vi "Temp.vi"() -> ()   [LabVIEW 2009]
uses:
  <vilib>/Platform/TimedLoop/XDataNode/XDataNode.xnode
  <vilib>/Platform/TimedLoop/XDataNode/loadlvalarms.vi
  <vilib>/Platform/TimedLoop/XDataNode/timing_clust.ctl
  <vilib>/Platform/TimedLoop/XDataNode/nitl_modes.ctl
  <vilib>/Platform/TimedLoop/XDataNode/wakeup.ctl
  <vilib>/Platform/TimedLoop/XDataNode/XDNodeRunTimeDep.lvlib
  <vilib>/Analysis/NI_AALBase.lvlib
  <vilib>/Analysis/NI_AALPro.lvlib
panel:
  out "time":dbl[](array[numeric])
  out "bearing":dbl[](array[numeric])
  out "XY Graph":cluster{dbl[], dbl[]}(graph)
  in  "Buffer Dimension":i32=10
  out "Iteration Duration 2":i64
  out "appended array":dbl[](array[numeric])
  in  "Simulate?":bool=TRUE
  out "Iteration Duration":i64=996
  in  "Prediction Time (s)":dbl=1.0
  out "Target Bearing":dbl
  in  "Sampling Time":dbl[](array[numeric])
  in  "Bearing History":dbl[](array[numeric])
  out "Bearing Sample":dbl=191.29579607174375 format="%0.2f"
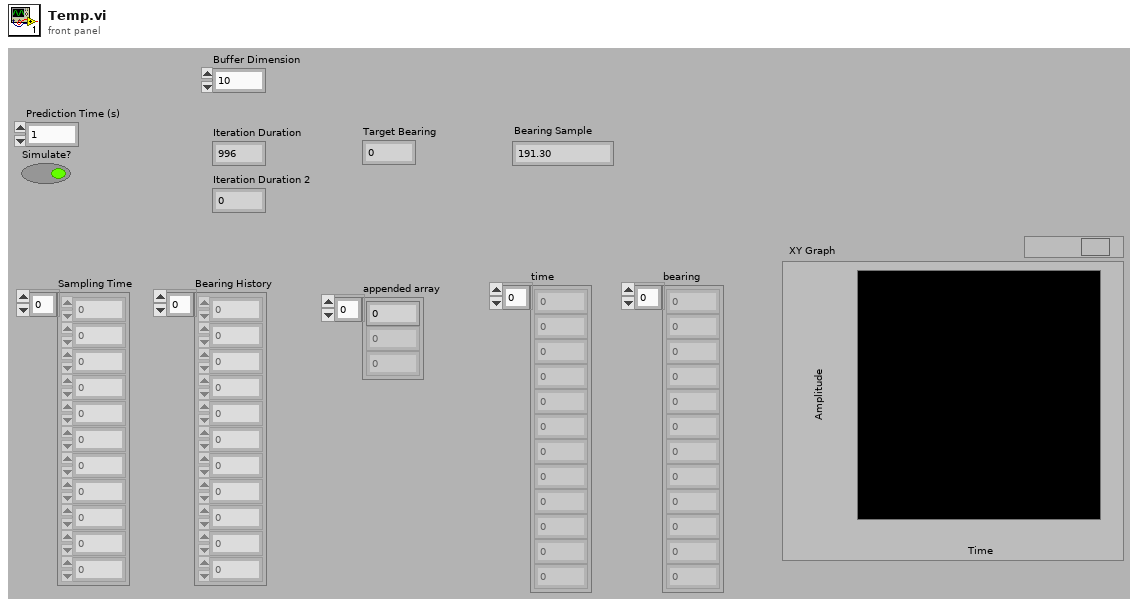
[diagram p1: front panel]
types:
  T1 = typedef "XDNodeRunTimeDep.lvlib/timing_clust.ctl" = cluster{"Expected End [f-1]":u64, "Actual End [f-1]":u64, "Finished Late? [f-1]":bool, "Expected End [i-1]":u64, "Actual End [i-1]":u64, "Finished Late? [i-1]":bool, "Expected Start [i]":u64, "Actual Start [i]":u64, "Expected Start [f]":u64, "Actual Start [f]":u64, "Source Name":string, "Structure Name":string, "Period":i64, "Deadline":i64, "Offset":i64, "Start":i64, "Priority":i32, "Timeout":i32, "Mode":T2, "Wakeup Reason":T3, "Error":errorcluster, "Source Type":string, "Secondary Source Type":string, "Global End Time":u64, "Global Start Time":u64, "Frame Duration":u64, "Iteration Duration":u64, "Assigned CPU":i32, "I/O Scan Engine Mode":u32}
  T2 = typedef "XDNodeRunTimeDep.lvlib/nitl_modes.ctl" = enum32{"No Change", "Process missed periods, maintain original phase", "Discard missed periods, maintain original phase", "Process missed periods, ignore original phase", "Discard missed periods, ignore original phase"}
  T3 = typedef "XDNodeRunTimeDep.lvlib/wakeup.ctl" = enum32{"Normal", "Aborted", "Asynchronous wakeup", "Timing source error", "Timed loop error", "Timeout"}
  T4 = cluster{"Sampling Time":dbl[], "Bearing History":dbl[]}
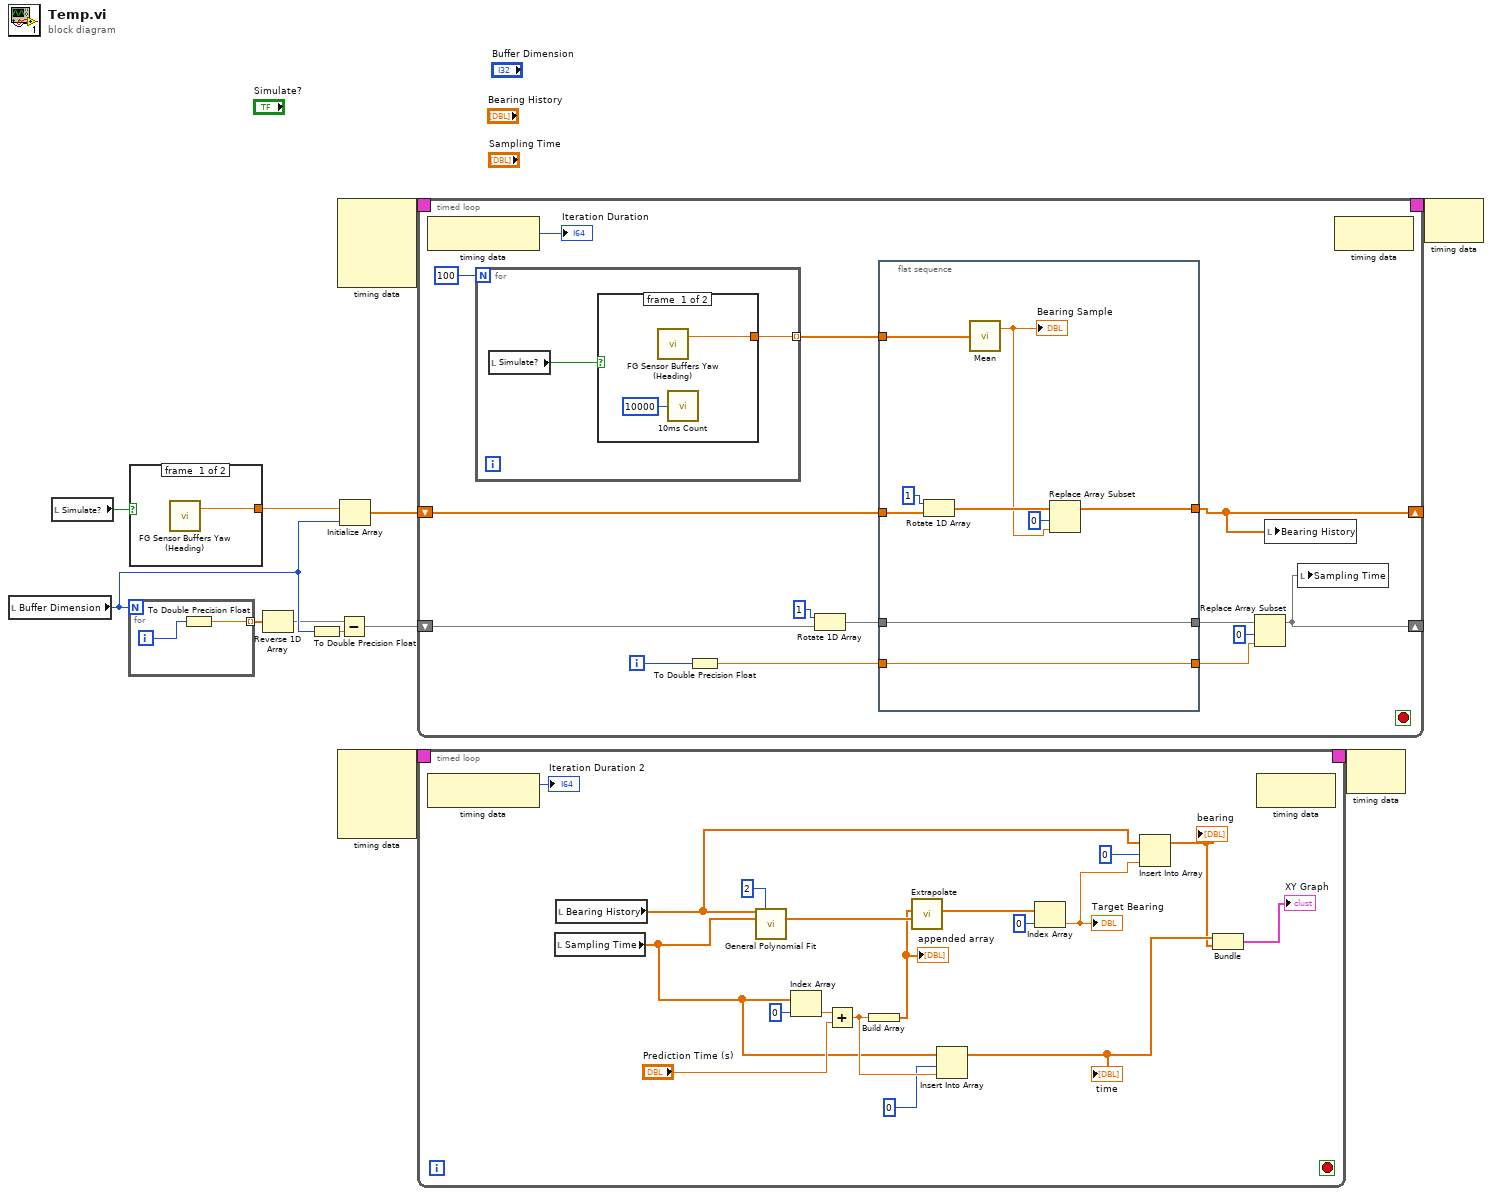
[diagram p0: block diagram]
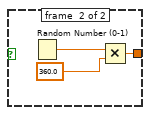
[diagram p2: hidden frame]
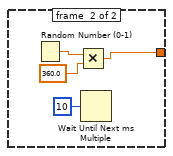
[diagram p3: hidden frame]
diagram:
  n1 = local read "Buffer Dimension"() -> (w4:i32)
  n2 = local read "Simulate?"() -> (w8:bool)
  n3 = for {
    N: w4 -> [_]
    tunnel: [w13] -> w5 mode=indexing
    i -> [w14]
    n4 = To Double Precision Float(number=w14) -> (double precision float=w13:dbl)
  }
  n5 = case shown="True" w8 {
    tunnel: [w15 w16] -> w7
    frame #0 {
      n6 = call "FG Sensor Buffers Yaw (Heading).vi"() -> ("Yaw Buffer Out"=w15:dbl)  [unwired: 3 in]
    }
    frame #1 {
      n7 = Random Number (0-1)() -> (number: 0 to 1=w17:dbl)
      n8 = Multiply(x=w17, y=360.0) -> (x*y=w16:dbl)
    }
  }
  n9 = Reverse 1D Array(array=w5) -> (reversed array=w1:dbl[])
  n10 = To Double Precision Float(number=w4) -> (double precision float=w2:dbl)
  n11 = node-c288() -> (w12:T1)  [unwired: 4 in]
  n12 = node-c288() -> (w10:T1)  [unwired: 4 in]
  n13 = Subtract(x=w1, y=w2) -> (x-y=w3:dbl[])
  n14 = Initialize Array(w7, w4) -> (w6:dbl[])
  n15 = timed-loop {
    timing: w12 -> [_]
    timing-out: [_] -> w11
    shift-right: [w20] -> _
    shift-left: w6 -> [w21]
    shift-right: [w19] -> _
    shift-left: w3 -> [w28]
    i -> [w30]
    stop <- _ stop-if-true
    n16 = node-c288() -> (→"Iteration Duration":i64)  [unwired: 1 in]
    n17 = for {
      N: 100 -> [_]
      tunnel: [w43] -> w31 mode=indexing
      n18 = local read "Simulate?"() -> (w42:bool)
      n19 = case shown="False" w42 {
        tunnel: [w44 w46] -> w43
        frame #0 {
          n20 = call "FG Sensor Buffers Yaw (Heading).vi"() -> ("Yaw Buffer Out"=w44:dbl)  [unwired: 3 in]
          n21 = call "10ms Count"("Count(uSec)"=u32 10000) -> ()  [unwired: 1 out]
        }
        frame #1 {
          n22 = Random Number (0-1)() -> (number: 0 to 1=w48:dbl)
          n23 = Multiply(x=w48, y=360.0) -> (x*y=w46:dbl)
          n24 = Wait Until Next ms Multiple(millisecond multiple=u32 10) -> ()  [unwired: 1 out]
        }
      }
    }
    n25 = To Double Precision Float(number=w30) -> (double precision float=w25:dbl)
    n26 = Rotate 1D Array(1:w28, 2:1 ("n")) -> (0:w26:dbl[])
    n27 = flat-sequence {
      tunnel: w31 -> [w41]
      tunnel: w26 -> [w40]
      tunnel: w25 -> [w39]
      tunnel: [w40] -> w23
      tunnel: [w39] -> w22
      tunnel: w21 -> [w37]
      tunnel: [w34] -> w20
      frame #0 {
        n28 = Rotate 1D Array(1:w37, 2:1 ("n")) -> (0:w35:dbl[])
        n29 = call <vilib>:"Mean.vi"("X"=w41) -> ("mean"=w33:dbl)  [unwired: 1 out]
        "Bearing Sample" <- w33
        n30 = Replace Array Subset(array=w35, new element=w33, index=0) -> (w34:dbl[])
      }
    }
    n31 = Replace Array Subset(array=w23, new element=w22, index=0) -> (w19:dbl[])
    n32 = local write "Bearing History"(w20) -> ()
    n33 = local write "Sampling Time"(w19) -> ()
    n34 = node-c288() -> ()  [unwired: 1 in, 1 out]
  }
  n35 = timed-loop {
    timing: w10 -> [_]
    timing-out: [_] -> w9
    stop <- _ stop-if-true
    n36 = node-c288() -> (→"Iteration Duration 2":i64)  [unwired: 1 in]
    n37 = local read "Sampling Time"() -> (w57:dbl[])
    n38 = local read "Bearing History"() -> (w60:dbl[])
    n39 = call <vilib>:"General Polynomial Fit.vi"("Y"=w60, "polynomial order"=2, "X"=w57) -> ("Polynomial Coefficients"=w69:dbl[])  [unwired: 9 in, 3 out]
    n40 = Index Array(array=w57, index=0) -> (element=w66:dbl)
    n41 = Add(x=w66, y="Prediction Time (s)") -> (x+y=w58:dbl)
    n42 = Build Array(w58) -> (w59:dbl[])
    "appended array" <- w59
    n43 = call "Extrapolate.vi"("Polynomial Coefficients"=w69, "xi"=w59) -> ("yi"=w68:dbl[])  [unwired: 9 in]
    n44 = Insert Into Array(array=w57, index=0, new element=w58) -> (w56:dbl[])
    "time" <- w56
    n45 = Index Array(array=w68, index=0) -> (element=w61:dbl)
    "Target Bearing" <- w61
    n46 = Insert Into Array(array=w60, index=0, new element=w61) -> (w55:dbl[])
    "bearing" <- w55
    n47 = Bundle("Sampling Time"=w56, "Bearing History"=w55) -> (→"XY Graph":T4)  [unwired: 1 in]
    n48 = node-c288() -> ()  [unwired: 1 in, 1 out]
  }
  n49 = node-c288(w9) -> ()  [unwired: 1 out]
  n50 = node-c288(w11) -> ()  [unwired: 1 out]
